vi "CH1_Address_decoder_calibration.vi"(11 "Range IN":dbl) -> (0 "LB":dbl, 1 "HB":dbl, 2 "UB":dbl, 3 "MB":dbl)   [LabVIEW 2012]
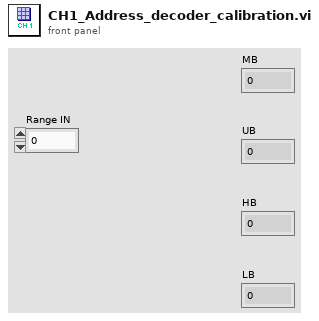
[diagram p1: front panel]
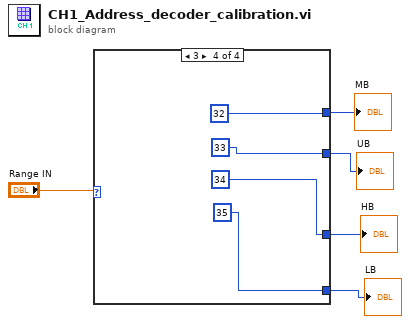
[diagram p0: block diagram]
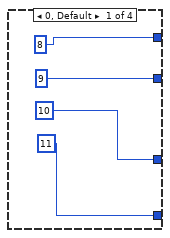
[diagram p2: hidden frame]
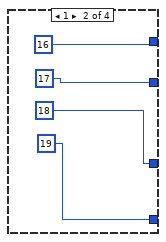
[diagram p3: hidden frame]
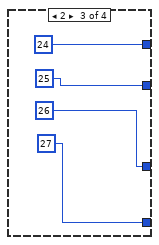
[diagram p4: hidden frame]
diagram:
  n1 = case shown="3" "Range IN" {
    tunnel: [8 16 24 32] -> w4
    tunnel: [9 17 25 33] -> w3
    tunnel: [10 18 26 34] -> w2
    tunnel: [11 19 27 35] -> w1
    frame 0, Default {
    }
    frame 1 {
    }
    frame 2 {
    }
    frame 3 {
    }
  }
  "LB" <- w1
  "MB" <- w4
  "UB" <- w3
  "HB" <- w2
